vi "kalman_filter.vi"() -> ()   [LabVIEW 2020]
uses:
  <vilib>/Analysis/Matrix/Datatypes/RealMatrix.ctl
  <vilib>/Analysis/baseanly.llb/Real A x B.vi
  <vilib>/Analysis/7linalg.llb/Real Transpose Matrix.vi
  <vilib>/Analysis/Matrix/Numeric/Add/Add - RM,RM.vi
  <vilib>/Analysis/baseanly.llb/Real Inverse Matrix.vi
  <vilib>/Analysis/Matrix/Numeric/Subtract/Subtract - RM,RM.vi
  <vilib>/Analysis/NI_AALPro.lvlib
  <vilib>/Analysis/NI_AALBase.lvlib
  <vilib>/Analysis/Matrix/NI_Matrix.lvlib
panel:
  out "phat":T1
  out "xhat":T1
  in  "y":T1
  in  "u":T1
  in  "B":T1
  in  "R":T1
  in  "C":T1
  in  "Q":T1
  in  "A":T1
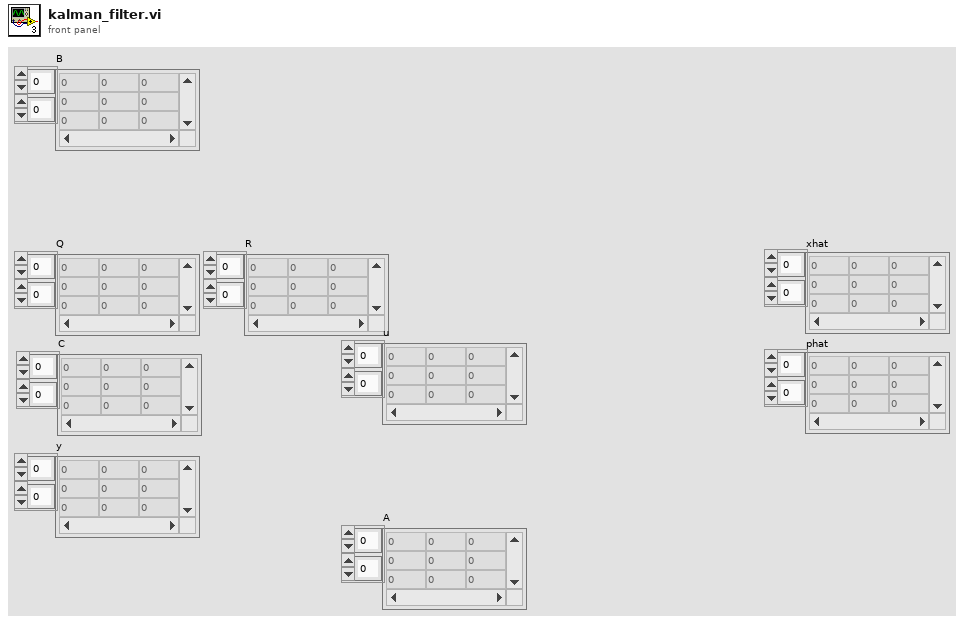
[diagram p1: front panel]
types:
  T1 = typedef "NI_Matrix.lvlib/RealMatrix.ctl" = dbl[][]
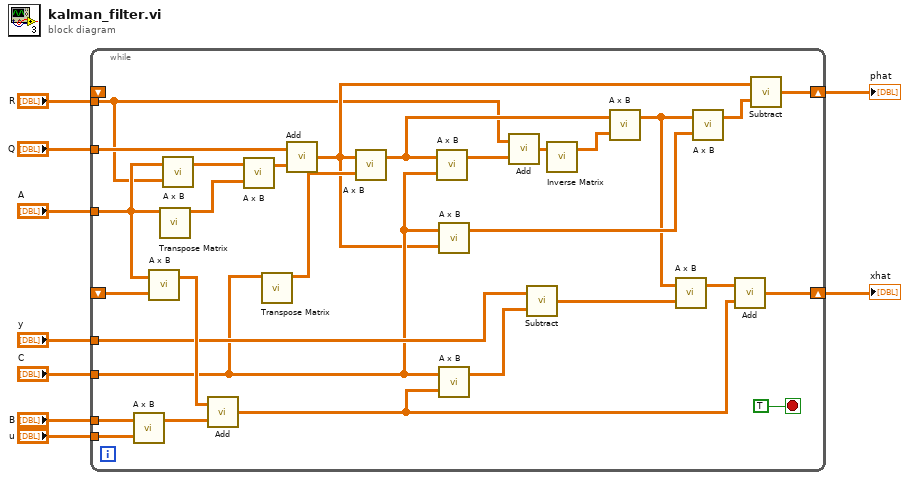
[diagram p0: block diagram]
diagram:
  n1 = while {
    shift-right: [w22] -> w2
    shift-left: _ -> [w14]
    tunnel: "y" -> [w20]
    tunnel: "B" -> [w19]
    tunnel: "u" -> [w18]
    tunnel: "R" -> [w10]
    tunnel: "C" -> [w17]
    tunnel: "Q" -> [w16]
    tunnel: "A" -> [w15]
    shift-right: [w11] -> w1
    shift-left: _ -> [_]
    stop <- TRUE stop-if-true
    n2 = call-poly <vilib>:"A x B.vi"("B"=w18, "A"=w19) -> ("A x B"=w25:T1)  [unwired: 1 out]
    n3 = call-poly <vilib>:"A x B.vi"("B"=w14, "A"=w15) -> ("A x B"=w21:T1)  [unwired: 1 out]
    n4 = call-poly <vilib>:"Transpose Matrix.vi"("Input Matrix"=w15) -> ("Matrix Transpose"=w37:T1)  [unwired: 9 in, 1 out]
    n5 = call-poly <vilib>:"A x B.vi"("B"=w10, "A"=w15) -> ("A x B"=w38:T1)  [unwired: 1 out]
    n6 = call-poly <vilib>:"Add.vi"("Real Matrix B"=w25, "Real Matrix A"=w21) -> ("A + B"=w24:T1)
    n7 = call-poly <vilib>:"A x B.vi"("B"=w37, "A"=w38) -> ("A x B"=w36:T1)  [unwired: 1 out]
    n8 = call-poly <vilib>:"Transpose Matrix.vi"("Input Matrix"=w17) -> ("Matrix Transpose"=w35:T1)  [unwired: 9 in, 1 out]
    n9 = call-poly <vilib>:"Add.vi"("Real Matrix B"=w36, "Real Matrix A"=w16) -> ("A + B"=w12:T1)
    n10 = call-poly <vilib>:"A x B.vi"("B"=w35, "A"=w12) -> ("A x B"=w31:T1)  [unwired: 1 out]
    n11 = call-poly <vilib>:"A x B.vi"("B"=w17, "A"=w31) -> ("A x B"=w34:T1)  [unwired: 1 out]
    n12 = call-poly <vilib>:"A x B.vi"("B"=w12, "A"=w17) -> ("A x B"=w30:T1)  [unwired: 1 out]
    n13 = call-poly <vilib>:"A x B.vi"("B"=w24, "A"=w17) -> ("A x B"=w29:T1)  [unwired: 1 out]
    n14 = call-poly <vilib>:"Add.vi"("Real Matrix B"=w34, "Real Matrix A"=w10) -> ("A + B"=w33:T1)
    n15 = call-poly <vilib>:"Subtract.vi"("Real Matrix B"=w29, "Real Matrix A"=w20) -> ("A - B"=w28:T1)
    n16 = call-poly <vilib>:"Inverse Matrix.vi"("Input Matrix"=w33) -> ("Inverse Matrix"=w32:T1)  [unwired: 1 in, 1 out]
    n17 = call-poly <vilib>:"A x B.vi"("B"=w32, "A"=w31) -> ("A x B"=w27:T1)  [unwired: 1 out]
    n18 = call-poly <vilib>:"A x B.vi"("B"=w28, "A"=w27) -> ("A x B"=w26:T1)  [unwired: 1 out]
    n19 = call-poly <vilib>:"A x B.vi"("B"=w30, "A"=w27) -> ("A x B"=w13:T1)  [unwired: 1 out]
    n20 = call-poly <vilib>:"Add.vi"("Real Matrix B"=w24, "Real Matrix A"=w26) -> ("A + B"=w22:T1)
    n21 = call-poly <vilib>:"Subtract.vi"("Real Matrix B"=w13, "Real Matrix A"=w12) -> ("A - B"=w11:T1)
  }
  "xhat" <- w2
  "phat" <- w1
